vi "_builtins_icon_create.vi"(10 "owner image":T1, 11 "icon":T2={"fg"=0, "bg"=16777215, "glyph"=enum."none", "header"={"text"="", "fg"=0, "bg"=16777215, "justify"=enum."center", "owner"=FALSE}, "text"={"text"=[], "fg"=0, "justify"=enum."center"}}) -> (3 "Image Data":T1)   [LabVIEW 2019, in "Script.lvlib"]
doc: "Creates a new flattened icon.\n\nCreated by: Ryan Pacini"
uses:
  Script.lvlib
  _builtins_icon.ctl
  <vilib>/picture/picture.llb/imagedata.ctl
panel:
  out "preview":picture
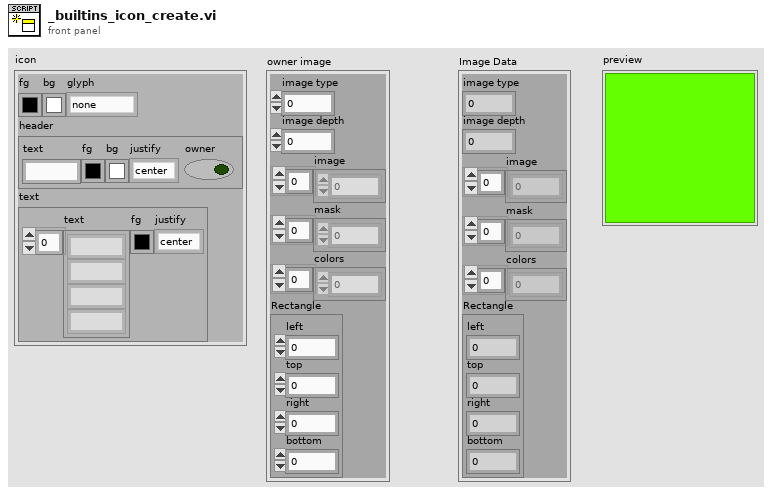
[diagram p1: front panel]
types:
  T1 = typedef "imagedata.ctl" = cluster{"image type":i32, "image depth":i32, "image":u8[], "mask":u8[], "colors":u32[], "Rectangle":cluster{"left":i16, "top":i16, "right":i16, "bottom":i16}}
  T2 = typedef "Script.lvlib/_builtins_icon.ctl" = cluster{"fg":u32, "bg":u32, "glyph":enum8{"none", "get", "set", "create", "config", "read", "write", "cmd", "tlm", "destroy", "ctl", "ctl_cmd", "ctl_tlm"}, "header":cluster{"text":string, "fg":u32, "bg":u32, "justify":enum8{"center", "left", "right"}, "owner":bool}, "text":cluster{"text":string[], "fg":u32, "justify":enum8{"center", "left", "right"}}}
  T3 = enum8{"none", "get", "set", "create", "config", "read", "write", "cmd", "tlm", "destroy", "ctl", "ctl_cmd", "ctl_tlm"}
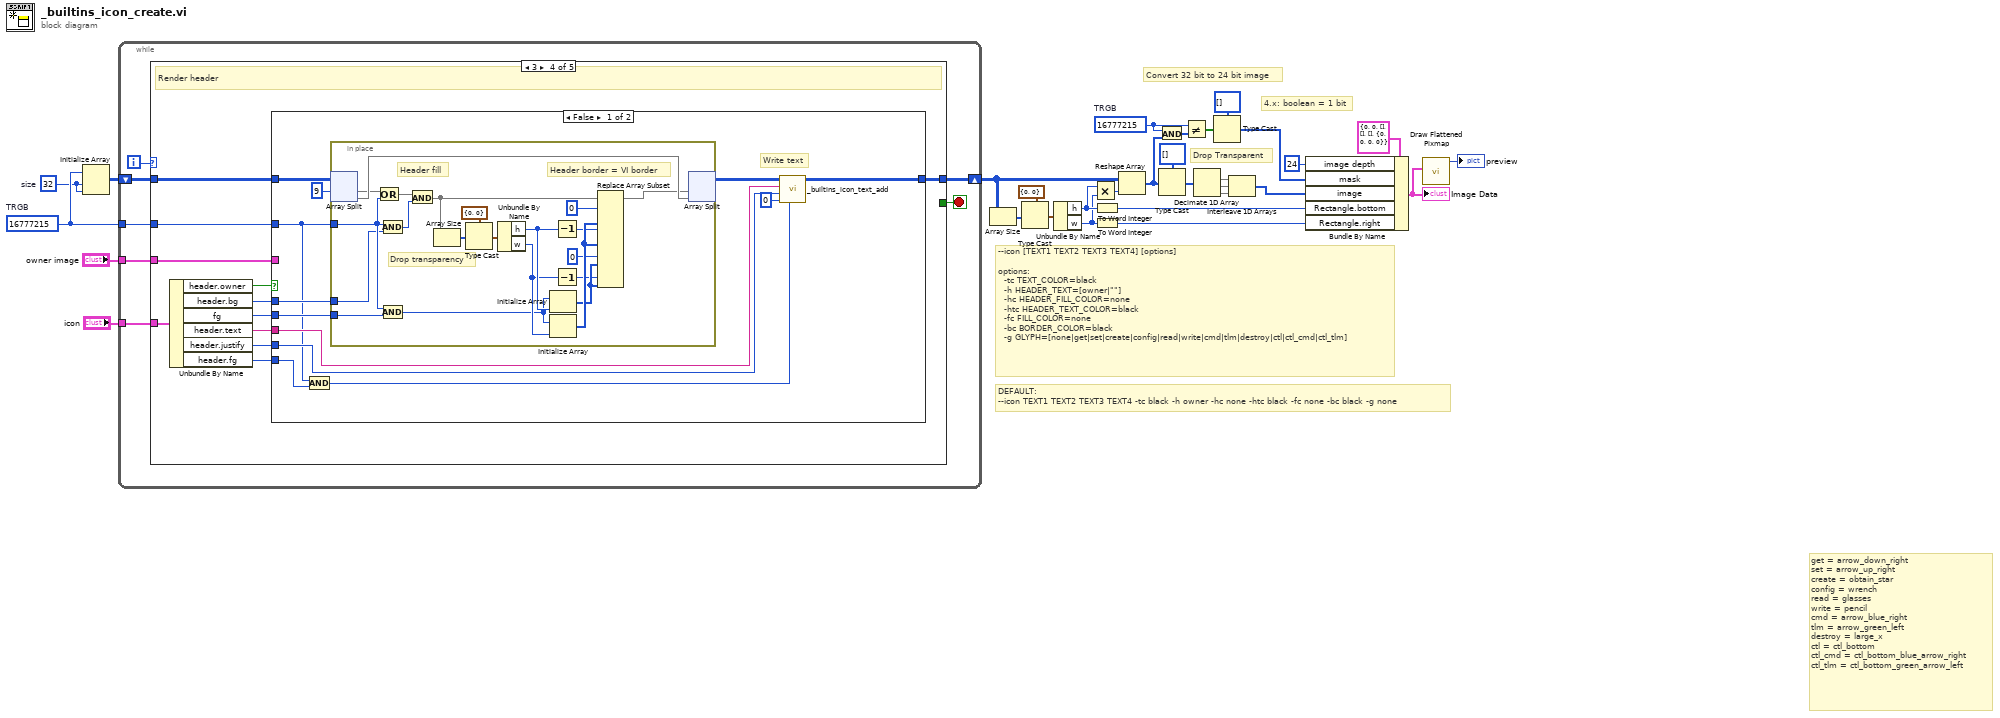
[diagram p0: block diagram]
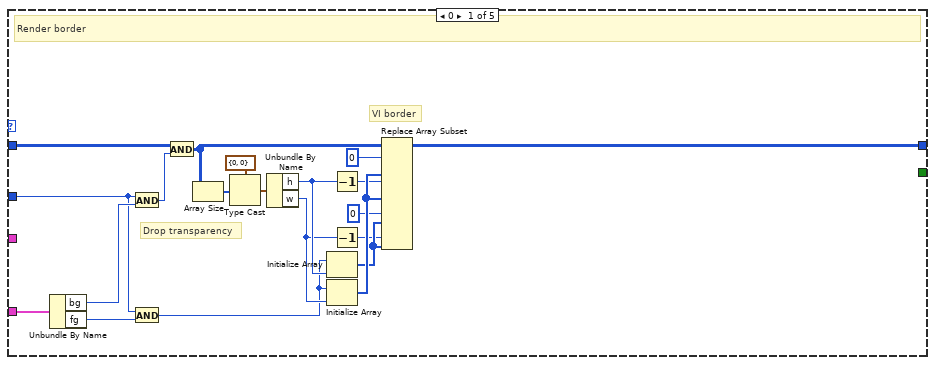
[diagram p2: hidden frame]
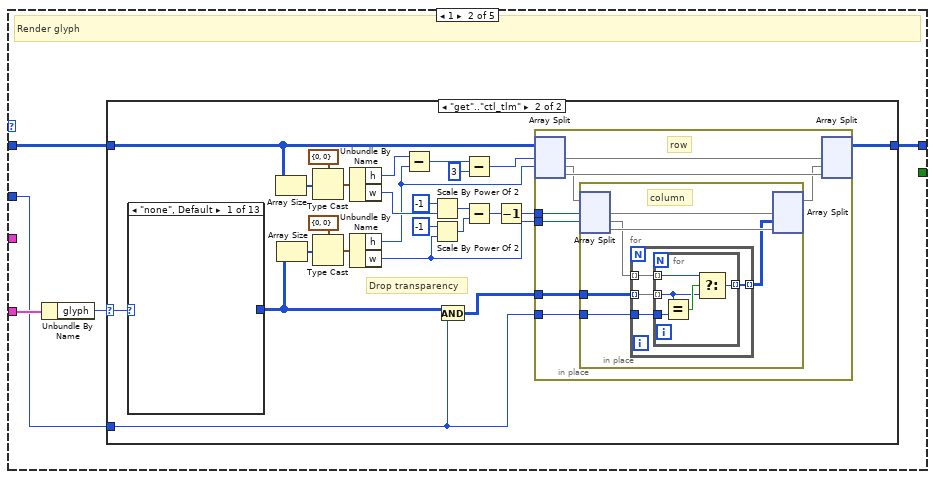
[diagram p3: hidden frame]
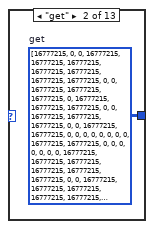
[diagram p5: hidden frame]
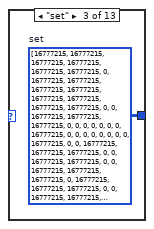
[diagram p6: hidden frame]
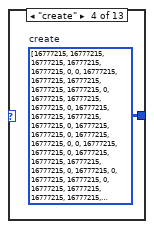
[diagram p7: hidden frame]
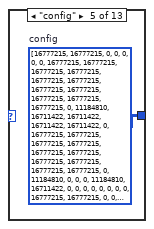
[diagram p8: hidden frame]
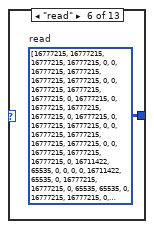
[diagram p9: hidden frame]
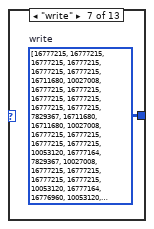
[diagram p10: hidden frame]
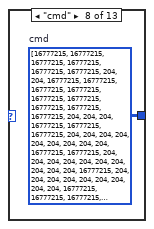
[diagram p11: hidden frame]
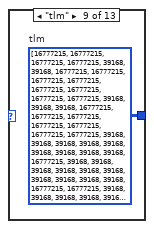
[diagram p12: hidden frame]
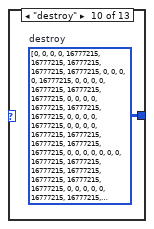
[diagram p13: hidden frame]
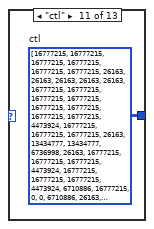
[diagram p14: hidden frame]
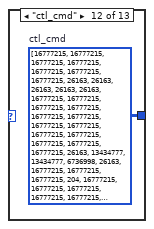
[diagram p15: hidden frame]
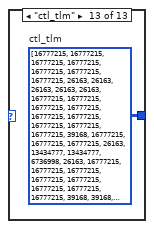
[diagram p16: hidden frame]
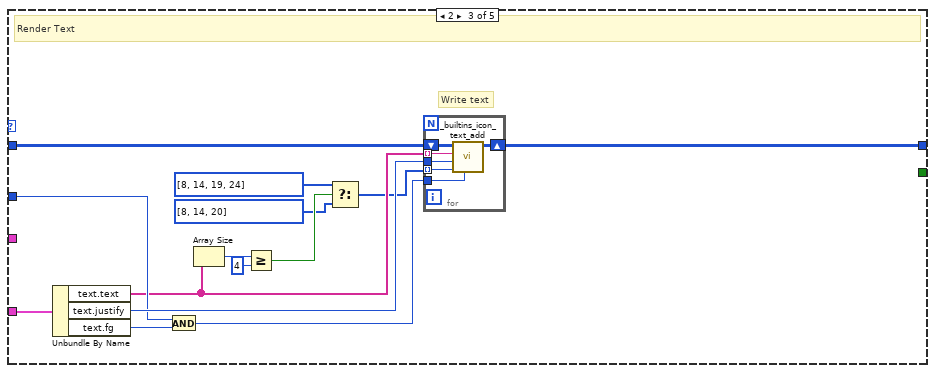
[diagram p17: hidden frame]
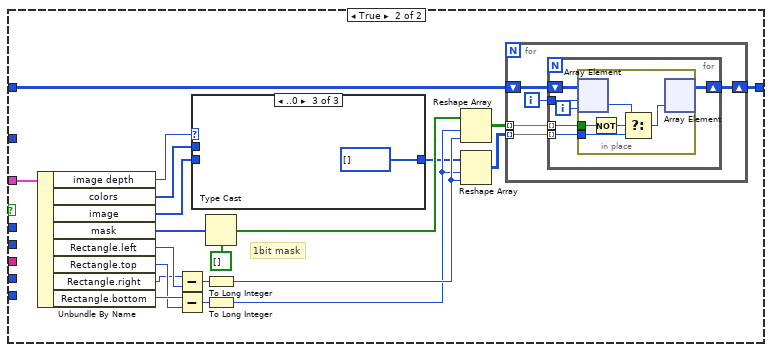
[diagram p18: hidden frame]
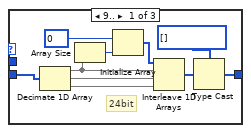
[diagram p19: hidden frame]
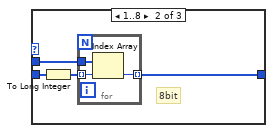
[diagram p20: hidden frame]
diagram:
  w5 = u32 16777215  # TRGB
  w27 = 32  # size
  w28 = u32 16777215  # TRGB
  # "Drop Transparent"
  # "4.x: boolean = 1 bit"
  # "Convert 32 bit to 24 bit image"
  # "DEFAULT:\n--icon TEXT1 TEXT2 TEXT3 TEXT4 -tc black -h owner -hc none -htc black -fc none -bc black -g none"
  # "get = arrow_down_right\nset = arrow_up_right\ncreate = obtain_star\nconfig = wrench\nread = glasses\nwrite = pencil\ncmd = arrow_blue_right\ntlm = arrow_green_left\ndestroy = large_x\nctl = ctl_bottom\nctl_cmd = ctl_bottom_blue_arrow_right\nctl_tlm = ctl_bottom_green_arrow_left"
  # "--icon [TEXT1 TEXT2 TEXT3 TEXT4] [options]\n\noptions:\n  -tc TEXT_COLOR=black\n  -h HEADER_TEXT=[owner|\"\"]\n  -hc HEADER_FILL_COLOR=none\n  -htc HEADER_TEXT_COLOR=black\n  -fc FILL_COLOR=none\n  -bc BORDER_COLOR=black\n  -g GLYPH=[none|get|set|create|config|read|write|cmd|tlm|destroy|ctl|ctl_cmd|ctl_tlm]"
  n1 = Initialize Array(w28, w27, w27) -> (w26:u32[][])
  n2 = while {
    shift-right: [w33] -> w24
    shift-left: w26 -> [w37]
    tunnel: "icon" -> [w34]
    tunnel: w28 -> [w32]
    tunnel: "owner image" -> [w31]
    i -> [w36]
    stop <- w35 stop-if-true
    n3 = case shown="3" w36 {
      tunnel: [w49 w59 w136 w150 w243] -> w33
      tunnel: w37 -> [w50 w60 w131 w153 w243]
      tunnel: [_ _ _ _ TRUE] -> w35
      tunnel: w34 -> [w57 w62 w137 w154 _]
      tunnel: w32 -> [w38 w58 w132 w146 _]
      tunnel: w31 -> [_ _ _ w144 _]
      frame 0 {
        # "VI border"
        # "Drop transparency"
        # "Render border"
        n4 = Unbundle By Name(w57) -> ("bg"=w42:u32, "fg"=w40:u32)
        n5 = And(x=w38, y=w42) -> (x .and. y?=w41:u32)
        n6 = And(x=w38, y=w40) -> (x .and. y?=w39:u32)
        n7 = And(x=w50, y=w41) -> (x .and. y?=w48:u32[][])
        n8 = Array Size(array=w48) -> (size(s)=w47:i32[])
        n9 = Type Cast(type=cluster{"h":i32, "w":i32} {"h"=0, "w"=0} ("size"), x=w47) -> (*(type *) &x=w45:cluster{"h":i32, "w":i32})
        n10 = Unbundle By Name(w45) -> ("h"=w44:i32, "w"=w43:i32)
        n11 = Initialize Array(w39, w44) -> (w54:u32[])
        n12 = Initialize Array(w39, w43) -> (w55:u32[])
        n13 = Decrement(x=w44) -> (x-1=w53:i32)
        n14 = Decrement(x=w43) -> (x-1=w52:i32)
        n15 = Replace Array Subset(array=w48, new element #1=w55, index (row) #1=0 ("index (row)"), new element #2=w55, index (row) #2=w53, new element #3=w54, index (col) #3=0 ("disabled index (col)"), new element #4=w54, index (col) #4=w52) -> (w49:u32[][])  [unwired: 4 in]
      }
      frame 1 {
        # "Render glyph"
        n16 = Unbundle By Name(w62) -> ("glyph"=w61:T3)
        n17 = case shown="\"get\"..\"ctl_tlm\"" w61 {
          selector: w61 -> [_ w65]
          tunnel: w60 -> [w63 w79]
          tunnel: [w63 w78] -> w59
          tunnel: w58 -> [_ w68]
          frame "none" {
          }
          frame "get".."ctl_tlm" {
            # "Drop transparency"
            n18 = case shown="\"none\", Default" w65 {
              tunnel: [_ w89 w90 w91 w92 w93 w94 w95 w96 w97 w98 w99 w100] -> w64
              frame "none", Default {
              }
              frame "get" {
                w89 = u32[][] [[16777215, 0, 0, 16777215, 16777215, 16777215, 16777215, 16777215, 16777215], [16777215, 0, 0, 16777215, 16777215, 16777215, 0, 16777215, 16777215], [16777215, 0, 0, 16777215, 16777215, 16777215, 0, 0, 16777215], [16777215, 0, 0, 0, 0, 0, 0, 0, 0], [16777215, 16777215, 0, 0, 0, 0, 0, 0, 0], [16777215, 16777215, 16777215, 16777215, 16777215, 16777215, 0, 0, 16777215], [16777215, 16777215, 16777215, 16777215, 16777215, 16777215, 0, 16777215, 16777215]]  # get
              }
              frame "set" {
                w90 = u32[][] [[16777215, 16777215, 16777215, 16777215, 16777215, 16777215, 0, 16777215, 16777215], [16777215, 16777215, 16777215, 16777215, 16777215, 16777215, 0, 0, 16777215], [16777215, 16777215, 0, 0, 0, 0, 0, 0, 0], [16777215, 0, 0, 0, 0, 0, 0, 0, 0], [16777215, 0, 0, 16777215, 16777215, 16777215, 0, 0, 16777215], [16777215, 0, 0, 16777215, 16777215, 16777215, 0, 16777215, 16777215], [16777215, 0, 0, 16777215, 16777215, 16777215, 16777215, 16777215, 16777215]]  # set
              }
              frame "create" {
                w91 = u32[][] [[16777215, 16777215, 16777215, 16777215, 16777215, 0, 0, 16777215, 16777215, 16777215, 16777215], [16777215, 0, 16777215, 16777215, 16777215, 0, 16777215, 16777215, 16777215, 16777215, 0], [16777215, 16777215, 0, 16777215, 16777215, 0, 0, 16777215, 16777215, 0, 16777215], [16777215, 16777215, 16777215, 0, 16777215, 0, 16777215, 16777215, 0, 16777215, 16777215], [16777215, 16777215, 16777215, 16777215, 16777215, 0, 0, 16777215, 16777215, 16777215, 16777215], [0, 0, 0, 0, 0, 0, 16777215, 0, 0, 0, 0], [0, 16777215, 0, 16777215, 0, 16777215, 0, 16777215, 0, 16777215, 0], [16777215, 16777215, 16777215, 16777215, 16777215, 0, 16777215, 16777215, 16777215, 16777215, 16777215], [16777215, 16777215, 16777215, 0, 16777215, 0, 0, 16777215, 0, 16777215, 16777215], [16777215, 16777215, 0, 16777215, 16777215, 0, 16777215, 16777215, 16777215, 0, 16777215], [16777215, 0, 16777215, 16777215, 16777215, 0, 0, 16777215, 16777215, 16777215, 0]]  # create
              }
              frame "config" {
                w92 = u32[][] [[16777215, 16777215, 0, 0, 0, 0, 0, 16777215, 16777215, 16777215, 16777215, 16777215, 16777215, 16777215, 16777215, 16777215, 16777215], [16777215, 0, 11184810, 16711422, 16711422, 16711422, 16711422, 0, 16777215, 16777215, 16777215, 16777215, 16777215, 16777215, 16777215, 16777215, 16777215], [16777215, 0, 11184810, 0, 0, 0, 11184810, 16711422, 0, 0, 0, 0, 0, 0, 0, 0, 16777215], [16777215, 0, 0, 16777215, 16777215, 0, 11184810, 11184810, 16711422, 16711422, 16711422, 16711422, 16711422, 16711422, 16711422, 16711422, 0], [16777215, 16777215, 16777215, 16777215, 16777215, 16777215, 0, 11184810, 11184810, 11184810, 11184810, 11184810, 11184810, 11184810, 11184810, 11184810, 0], [16777215, 0, 0, 16777215, 16777215, 0, 11184810, 11184810, 7829367, 7829367, 7829367, 7829367, 7829367, 7829367, 7829367, 7829367, 0], [16777215, 0, 7829367, 0, 0, 0, 11184810, 7829367, 0, 0, 0, 0, 0, 0, 0, 0, 16777215], [16777215, 0, 7829367, 7829367, 7829367, 7829367, 7829367, 0, 16777215, 16777215, 16777215, 16777215, 16777215, 16777215, 16777215, 16777215, 16777215], [16777215, 16777215, 0, 0, 0, 0, 0, 16777215, 16777215, 16777215, 16777215, 16777215, 16777215, 16777215, 16777215, 16777215, 16777215]]  # config
              }
              frame "read" {
                w93 = u32[][] [[16777215, 16777215, 16777215, 16777215, 0, 0, 16777215, 16777215, 16777215, 16777215, 0, 0], [16777215, 16777215, 16777215, 0, 16777215, 0, 16777215, 16777215, 16777215, 0, 16777215, 0], [16777215, 16777215, 0, 0, 16777215, 16777215, 16777215, 16777215, 0, 0, 16777215, 16777215], [16777215, 0, 16711422, 65535, 0, 0, 0, 0, 16711422, 65535, 0, 16777215], [16777215, 0, 65535, 65535, 0, 16777215, 16777215, 0, 65535, 65535, 0, 16777215], [16777215, 16777215, 0, 0, 16777215, 16777215, 16777215, 16777215, 0, 0, 16777215, 16777215]]  # read
              }
              frame "write" {
                w94 = u32[][] [[16777215, 16777215, 16777215, 16777215, 16777215, 16777215, 16711680, 10027008, 16777215], [16777215, 16777215, 16777215, 16777215, 16777215, 7829367, 16711680, 16711680, 10027008], [16777215, 16777215, 16777215, 16777215, 10053120, 16777164, 7829367, 10027008, 16777215], [16777215, 16777215, 16777215, 10053120, 16777164, 16776960, 10053120, 16777215, 16777215], [16777215, 16777215, 10053120, 16777164, 16776960, 10053120, 16777215, 16777215, 16777215], [16777215, 3342336, 13421619, 13421619, 10053120, 16777215, 16777215, 16777215, 16777215], [16777215, 3342336, 3342336, 16777215, 16777215, 16777215, 16777215, 16777215, 16777215]]  # write
              }
              frame "cmd" {
                w95 = u32[][] [[16777215, 16777215, 16777215, 16777215, 16777215, 16777215, 204, 204, 16777215, 16777215, 16777215], [16777215, 16777215, 16777215, 16777215, 16777215, 16777215, 204, 204, 204, 16777215, 16777215], [16777215, 204, 204, 204, 204, 204, 204, 204, 204, 204, 16777215], [16777215, 204, 204, 204, 204, 204, 204, 204, 204, 204, 204], [16777215, 204, 204, 204, 204, 204, 204, 204, 204, 204, 16777215], [16777215, 16777215, 16777215, 16777215, 16777215, 16777215, 204, 204, 204, 16777215, 16777215], [16777215, 16777215, 16777215, 16777215, 16777215, 16777215, 204, 204, 16777215, 16777215, 16777215]]  # cmd
              }
              frame "tlm" {
                w96 = u32[][] [[16777215, 16777215, 16777215, 16777215, 39168, 39168, 16777215, 16777215, 16777215, 16777215, 16777215], [16777215, 16777215, 16777215, 39168, 39168, 39168, 16777215, 16777215, 16777215, 16777215, 16777215], [16777215, 16777215, 39168, 39168, 39168, 39168, 39168, 39168, 39168, 39168, 39168], [16777215, 39168, 39168, 39168, 39168, 39168, 39168, 39168, 39168, 39168, 39168], [16777215, 16777215, 39168, 39168, 39168, 39168, 39168, 39168, 39168, 39168, 39168], [16777215, 16777215, 16777215, 39168, 39168, 39168, 16777215, 16777215, 16777215, 16777215, 16777215], [16777215, 16777215, 16777215, 16777215, 39168, 39168, 16777215, 16777215, 16777215, 16777215, 16777215]]  # tlm
              }
              frame "destroy" {
                w97 = u32[][] [[0, 0, 0, 0, 16777215, 16777215, 16777215, 16777215, 16777215, 0, 0, 0, 0], [16777215, 0, 0, 0, 0, 16777215, 16777215, 16777215, 0, 0, 0, 0, 16777215], [16777215, 16777215, 0, 0, 0, 0, 16777215, 0, 0, 0, 0, 16777215, 16777215], [16777215, 16777215, 16777215, 0, 0, 0, 0, 0, 0, 0, 16777215, 16777215, 16777215], [16777215, 16777215, 16777215, 16777215, 0, 0, 0, 0, 0, 16777215, 16777215, 16777215, 16777215], [16777215, 16777215, 16777215, 16777215, 0, 0, 0, 0, 0, 16777215, 16777215, 16777215, 16777215], [16777215, 16777215, 16777215, 0, 0, 0, 0, 0, 0, 0, 16777215, 16777215, 16777215], [16777215, 16777215, 0, 0, 0, 0, 16777215, 0, 0, 0, 0, 16777215, 16777215], [16777215, 0, 0, 0, 0, 16777215, 16777215, 16777215, 0, 0, 0, 0, 16777215], [0, 0, 0, 0, 16777215, 16777215, 16777215, 16777215, 16777215, 0, 0, 0, 0]]  # destroy
              }
              frame "ctl" {
                w98 = u32[][] [[16777215, 16777215, 16777215, 16777215, 16777215, 16777215, 26163, 26163, 26163, 26163, 26163, 16777215, 16777215, 16777215, 16777215, 16777215, 16777215], [16777215, 16777215, 4473924, 16777215, 16777215, 16777215, 26163, 13434777, 13434777, 6736998, 26163, 16777215, 16777215, 16777215, 4473924, 16777215, 16777215], [16777215, 4473924, 6710886, 16777215, 0, 0, 6710886, 26163, 13434777, 26163, 6710886, 0, 0, 16777215, 6710886, 4473924, 16777215], [4473924, 6710886, 6710886, 16777215, 0, 10066329, 10066329, 26163, 6736998, 26163, 10066329, 10066329, 0, 16777215, 6710886, 6710886, 4473924], [16777215, 10066329, 6710886, 16777215, 0, 0, 0, 6710886, 6736998, 6710886, 0, 0, 0, 16777215, 6710886, 10066329, 16777215], [16777215, 16777215, 10066329, 16777215, 16777215, 10066329, 16777215, 16777215, 26163, 16777215, 16777215, 10066329, 16777215, 16777215, 10066329, 16777215, 16777215]]  # ctl
              }
              frame "ctl_cmd" {
                w99 = u32[][] [[16777215, 16777215, 16777215, 16777215, 16777215, 16777215, 16777215, 26163, 26163, 26163, 26163, 26163, 16777215, 16777215, 16777215, 16777215, 16777215, 16777215], [16777215, 16777215, 16777215, 16777215, 16777215, 16777215, 16777215, 26163, 13434777, 13434777, 6736998, 26163, 16777215, 16777215, 16777215, 204, 16777215, 16777215], [16777215, 16777215, 16777215, 16777215, 16777215, 0, 0, 6710886, 26163, 13434777, 26163, 6710886, 0, 0, 16777215, 204, 204, 16777215], [16777215, 16777215, 16777215, 16777215, 16777215, 0, 10066329, 10066329, 26163, 6736998, 26163, 10066329, 10066329, 0, 16777215, 204, 204, 204], [16777215, 16777215, 16777215, 16777215, 16777215, 0, 0, 0, 6710886, 6736998, 6710886, 0, 0, 0, 16777215, 204, 204, 16777215], [16777215, 16777215, 16777215, 16777215, 16777215, 16777215, 10066329, 16777215, 16777215, 26163, 16777215, 16777215, 10066329, 16777215, 16777215, 204, 16777215, 16777215]]  # ctl_cmd
              }
              frame "ctl_tlm" {
                w100 = u32[][] [[16777215, 16777215, 16777215, 16777215, 16777215, 16777215, 16777215, 26163, 26163, 26163, 26163, 26163, 16777215, 16777215, 16777215, 16777215, 16777215, 16777215], [16777215, 16777215, 16777215, 39168, 16777215, 16777215, 16777215, 26163, 13434777, 13434777, 6736998, 26163, 16777215, 16777215, 16777215, 16777215, 16777215, 16777215], [16777215, 16777215, 39168, 39168, 16777215, 0, 0, 6710886, 26163, 13434777, 26163, 6710886, 0, 0, 16777215, 16777215, 16777215, 16777215], [16777215, 39168, 39168, 39168, 16777215, 0, 10066329, 10066329, 26163, 6736998, 26163, 10066329, 10066329, 0, 16777215, 16777215, 16777215, 16777215], [16777215, 16777215, 39168, 39168, 16777215, 0, 0, 0, 6710886, 6736998, 6710886, 0, 0, 0, 16777215, 16777215, 16777215, 16777215], [16777215, 16777215, 16777215, 39168, 16777215, 16777215, 10066329, 16777215, 16777215, 26163, 16777215, 16777215, 10066329, 16777215, 16777215, 16777215, 16777215, 16777215]]  # ctl_tlm
              }
            }
            n19 = Array Size(array=w79) -> (size(s)=w88:i32[])
            n20 = Array Size(array=w64) -> (size(s)=w83:i32[])
            n21 = Type Cast(type=cluster{"h":i32, "w":i32} {"h"=0, "w"=0} ("size"), x=w88) -> (*(type *) &x=w86:cluster{"h":i32, "w":i32})
            n22 = Type Cast(type=cluster{"h":i32, "w":i32} {"h"=0, "w"=0} ("size"), x=w83) -> (*(type *) &x=w85:cluster{"h":i32, "w":i32})
            n23 = Unbundle By Name(w86) -> ("h"=w77:i32, "w"=w80:i32)
            n24 = Unbundle By Name(w85) -> ("h"=w73:i32, "w"=w69:i32)
            n25 = Subtract(x=w77, y=w73) -> (x-y=w76:i32)
            n26 = Scale By Power Of 2(n=i16 -1, x=w80) -> (x*2^n=w71:i32)
            n27 = Scale By Power Of 2(n=i16 -1, x=w69) -> (x*2^n=w72:i32)
            n28 = And(x=w64, y=w68) -> (x .and. y?=w67:u32[][])
            n29 = Subtract(x=w76, y=3) -> (x-y=w74:i32)
            n30 = Subtract(x=w71, y=w72) -> (x-y=w70:i32)
            n31 = Decrement(x=w70) -> (x-1=w66:i32)
            n32 = in-place {
              in-place-border: w67 -> [w103]
              in-place-border: w66 -> [w105]
              in-place-border: w68 -> [w102]
              in-place-border: w69 -> [w101]
              # "row"
              n33 = in-place-split #1(w79, w74, w73) -> (w108:u32[][], w106:u32[][], w107:u32[][])
              n34 = in-place {
                in-place-border: w103 -> [w111]
                in-place-border: w102 -> [w110]
                # "column"
                n35 = in-place-split #2(w106, w105, w101) -> (w114:u32[][], w112:u32[][], w113:u32[][])
                n36 = for {
                  tunnel: w112 -> [w118] mode=indexing
                  tunnel: w111 -> [w117] mode=indexing
                  tunnel: w110 -> [w116]
                  tunnel: [w115] -> w109 mode=indexing
                  n37 = for {
                    tunnel: w118 -> [w121] mode=indexing
                    tunnel: w117 -> [w120] mode=indexing
                    tunnel: w116 -> [w123]
                    tunnel: [w119] -> w115 mode=indexing
                    n38 = Equal?(x=w120, y=w123) -> (x = y?=w122:bool)
                    n39 = Select(t=w121, s=w122, f=w120) -> (s? t:f=w119:u32)
                  }
                }
                n40 = in-place-split #2(w114, w109, w113) -> (w104:u32[][])  [unwired: 2 out]
              }
              n41 = in-place-split #1(w108, w104, w107) -> (w78:u32[][])  [unwired: 2 out]
            }
          }
        }
      }
      frame 2 {
        # "Write text"
        # "Render Text"
        n42 = Unbundle By Name(w137) -> ("text.text"=w130:string[], "text.justify"=w135:enum8{"center", "left", "right"}, "text.fg"=w134:u32)
        n43 = And(x=w132, y=w134) -> (x .and. y?=w133:u32)
        n44 = Array Size(array=w130) -> (size(s)=w129:i32)
        n45 = Greater Or Equal?(x=w129, y=4) -> (x >= y?=w127:bool)
        n46 = Select(t=i32[] [8, 14, 19, 24], s=w127, f=i32[] [8, 14, 20]) -> (s? t:f=w125:i32[])
        n47 = for {
          tunnel: w130 -> [w142] mode=indexing
          tunnel: w135 -> [w141]
          tunnel: w133 -> [w140]
          tunnel: w125 -> [w138] mode=indexing
          shift-right: [w143] -> w136
          shift-left: w131 -> [w139]
          n48 = call "_builtins_icon_text_add.vi"("Color"=w140, "Top"=w138, "Justify"=w141, "Text"=w142, "Image in"=w139) -> ("Image out"=w143:u32[][])  [unwired: 6 in]
        }
      }
      frame 3 {
        # "Render header"
        n49 = Unbundle By Name(w154) -> ("header.owner"=w145:bool, "header.bg"=w151:u32, "fg"=w152:u32, "header.text"=w149:string, "header.justify"=w148:enum8{"center", "left", "right"}, "header.fg"=w147:u32)
        n50 = case shown="False" w145 {
          tunnel: w153 -> [w166 w195]
          tunnel: w152 -> [w164 _]
          tunnel: w151 -> [w163 _]
          tunnel: [w161 w194] -> w150
          tunnel: w149 -> [w160 _]
          tunnel: w148 -> [w159 _]
          tunnel: w147 -> [w157 _]
          tunnel: w146 -> [w155 _]
          tunnel: w144 -> [_ w207]
          frame False {
            # "Write text"
            n51 = And(x=w155, y=w157) -> (x .and. y?=w156:u32)
            n52 = in-place {
              in-place-border: w155 -> [w172]
              in-place-border: w163 -> [w170]
              in-place-border: w164 -> [w168]
              # "Header fill"
              # "Header border = VI border"
              # "Drop transparency"
              n53 = in-place-split #3(w166, 9) -> (w173:u32[][], w174:u32[][])
              n54 = Or(x=w173, y=w172) -> (x .or. y?=w171:u32[][])
              n55 = And(x=w172, y=w170) -> (x .and. y?=w169:u32)
              n56 = And(x=w172, y=w168) -> (x .and. y?=w175:u32)
              n57 = And(x=w171, y=w169) -> (x .and. y?=w181:u32[][])
              n58 = Array Size(array=w181) -> (size(s)=w180:i32[])
              n59 = Type Cast(type=cluster{"h":i32, "w":i32} {"h"=0, "w"=0} ("size"), x=w180) -> (*(type *) &x=w178:cluster{"h":i32, "w":i32})
              n60 = Unbundle By Name(w178) -> ("h"=w177:i32, "w"=w176:i32)
              n61 = Initialize Array(w175, w177) -> (w185:u32[])
              n62 = Initialize Array(w175, w176) -> (w186:u32[])
              n63 = Decrement(x=w177) -> (x-1=w184:i32)
              n64 = Decrement(x=w176) -> (x-1=w183:i32)
              n65 = Replace Array Subset(array=w181, new element #1=w186, index (row) #1=0 ("index (row)"), new element #2=w186, index (row) #2=w184, new element #3=w185, index (col) #3=0 ("disabled index (col)"), new element #4=w185, index (col) #4=w183) -> (w167:u32[][])  [unwired: 4 in]
              n66 = in-place-split #3(w167, w174) -> (w162:u32[][])  [unwired: 1 out]
            }
            n67 = call "_builtins_icon_text_add.vi"("Color"=w156, "Top"=0, "Justify"=w159, "Text"=w160, "Image in"=w162) -> ("Image out"=w161:u32[][])  [unwired: 6 in]
          }
          frame True {
            # "1bit mask"
            n68 = Unbundle By Name(w207) -> ("image depth"=w189:i32, "colors"=w190:u32[], "image"=w191:u8[], "mask"=w200:u8[], "Rectangle.left"=w204:i16, "Rectangle.top"=w205:i16, "Rectangle.right"=w203:i16, "Rectangle.bottom"=w206:i16)
            n69 = Subtract(x=w203, y=w204) -> (x-y=w201:i16)
            n70 = Subtract(x=w206, y=w205) -> (x-y=w202:i16)
            n71 = case shown="..0" w189 {
              tunnel: w191 -> [w217 w221 _]
              tunnel: w190 -> [_ w219 _]
              tunnel: [w212 w218 u32[] []] -> w188
              frame 9.. {
                # "24bit"
                n72 = Decimate 1D Array(w217) -> (w210:u8[], w215:u8[], w216:u8[])
                n73 = Array Size(array=w210) -> (size(s)=w209:i32)
                n74 = Initialize Array(u8 0, w209) -> (w213:u8[])
                n75 = Interleave 1D Arrays(w213, w210, w215, w216) -> (w214:u8[])
                n76 = Type Cast(type=u32[] [], x=w214) -> (*(type *) &x=w212:u32[])
              }
              frame 1..8 {
                # "8bit"
                n77 = To Long Integer(number=w221) -> (32bit integer=w220:i32[])
                n78 = for {
                  tunnel: w220 -> [w224] mode=indexing
                  tunnel: w219 -> [w223]
                  tunnel: [w222] -> w218 mode=indexing
                  n79 = Index Array(array=w223, index=w224) -> (element=w222:u32)
                }
              }
              frame ..0 {
              }
            }
            n80 = Type Cast(type=bool[] [], x=w200) -> (*(type *) &x=w196:bool[])
            n81 = To Long Integer(number=w201) -> (32bit integer=w198:i32)
            n82 = To Long Integer(number=w202) -> (32bit integer=w197:i32)
            n83 = Reshape Array(w196, w197, w198) -> (w193:bool[][])
            n84 = Reshape Array(w188, w197, w198) -> (w192:u32[][])
            n85 = for {
              shift-right: [w229] -> w194
              shift-left: w195 -> [w230]
              tunnel: w193 -> [w227] mode=indexing
              tunnel: w192 -> [w226] mode=indexing
              i -> [w228]
              n86 = for {
                shift-right: [w234] -> w229
                shift-left: w230 -> [w236]
                tunnel: w228 -> [w235]
                tunnel: w227 -> [w232] mode=indexing
                tunnel: w226 -> [w231] mode=indexing
                i -> [w233]
                n87 = in-place {
                  in-place-border: w232 -> [w239]
                  in-place-border: w231 -> [w238]
                  n88 = in-place-array #4(w236, w235, w233) -> (w241:u32)
                  n89 = Not(x=w239) -> (.not. x?=w237:bool)
                  n90 = Select(t=w241, s=w237, f=w238) -> (s? t:f=w240:u32)
                  n91 = in-place-array #4(w240) -> (w234:u32[][])  [unwired: 2 out]
                }
              }
            }
          }
        }
      }
      frame Default {
      }
    }
  }
  n92 = Array Size(array=w24) -> (size(s)=w21:i32[])
  n93 = Type Cast(type=cluster{"h":i32, "w":i32} {"h"=0, "w"=0} ("size"), x=w21) -> (*(type *) &x=w19:cluster{"h":i32, "w":i32})
  n94 = Unbundle By Name(w19) -> ("h"=w16:i32, "w"=w15:i32)
  n95 = Multiply(x=w16, y=w15) -> (x*y=w14:i32)
  n96 = To Word Integer(number=w16) -> (16bit integer=w18:i16)
  n97 = To Word Integer(number=w15) -> (16bit integer=w17:i16)
  n98 = Reshape Array(w24, w14) -> (w7:u32[])
  n99 = And(x=w5, y=w7) -> (x .and. y?=w6:u32[])
  n100 = Type Cast(type=u8[] [], x=w7) -> (*(type *) &x=w10:u8[])
  n101 = Not Equal?(x=w5, y=w6) -> (x != y?=w4:bool[])
  n102 = Decimate 1D Array(w10) -> (w13:u8[], w12:u8[], w11:u8[])  [unwired: 1 out]
  n103 = Type Cast(type=u8[] [], x=w4) -> (*(type *) &x=w3:u8[])
  n104 = Interleave 1D Arrays(w13, w12, w11) -> (w9:u8[])
  n105 = Bundle By Name(cluster=T1 {"image type"=0, "image depth"=0, "image"=[], "mask"=[], "colors"=[], "Rectangle"={"left"=0, "top"=0, "right"=0, "bottom"=0}} ("Image Data"), "image depth"=24, "mask"=w3, "image"=w9, "Rectangle.bottom"=w18, "Rectangle.right"=w17) -> (w25:T1)
  "Image Data" <- w25
  n106 = call <vilib>:"Draw Flattened Pixmap.vi"("image data"=w25) -> ("new picture"=→"preview":picture)  [unwired: 8 in]
